vi "LJM_eNames2D.vi"(0 "Handle In":i32, 1 "NumFrames (Auto-Detect)":i32=-1, 5 "aNames":string[](array[string]), 9 "aValuesIn":dbl[][](array[numeric]) format="%.2f", 11 "error in":errorcluster, 12 "aWrites":i32[](array[ring]) items=["Read", "Write"], 13 "aNumValues":i32[](array[numeric])) -> (4 "Handle Out":i32, 10 "aValuesOut":dbl[][](array[numeric]) format="%.2f", 14 "ErrorAddress":i32, 15 "error out":errorcluster)   [LabVIEW 2020]
panel:
  # "1/20/2015:  Default value of NumFrames changed to -1 which\nequates to Auto-Detect.  If NumFrames = -1, then the NumFrames\ncontrol is ignored and the size of aNames/aAddresses is used to\ndetermine how many frames there are."
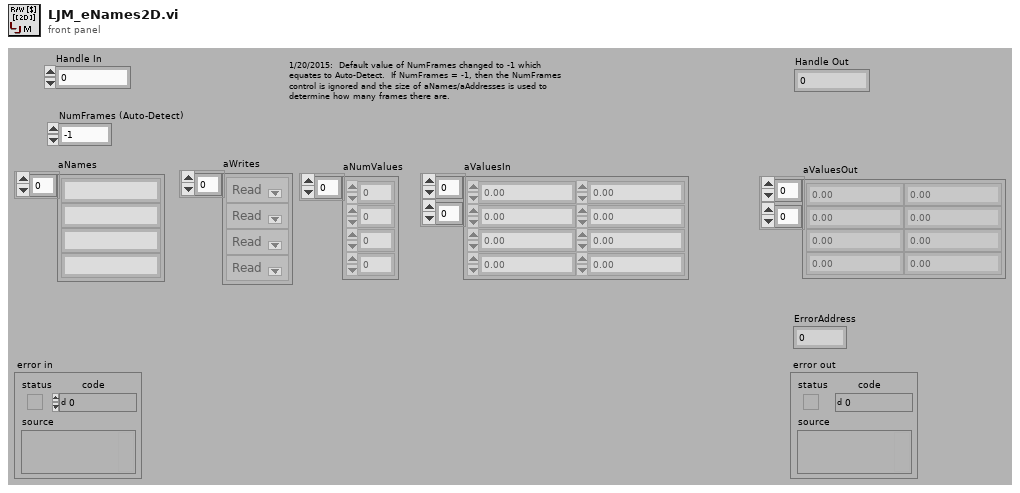
[diagram p1: front panel]
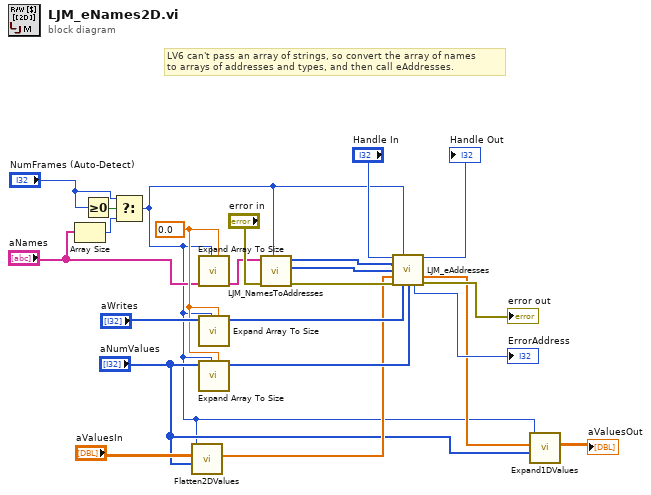
[diagram p0: block diagram]
diagram:
  w11 = 0.0 ("Default Value")
  # "LV6 can't pass an array of strings, so convert the array of names\nto arrays of addresses and types, and then call eAddresses."
  n1 = Array Size(array="aNames") -> (size(s)=w6:i32)
  n2 = Greater Or Equal To 0?(x="NumFrames (Auto-Detect)") -> (x >= 0?=w5:bool)
  n3 = Select(t="NumFrames (Auto-Detect)", s=w5, f=w6) -> (s? t:f=w1:i32)
  n4 = call "Flatten2DValues.vi"("NumValues"="aNumValues", "Values 2D"="aValuesIn", "NumFrames"=w1) -> ("Values 1D"=w8:dbl[])  [unwired: 8 in]
  n5 = call "Expand Array To Size.vi"("Default Value"=w11, "# Elements"=w1, "String Array In"="aNames") -> ("String Array Out"=w21:string[])  [unwired: 4 in, 4 out]
  n6 = call "Expand Array To Size.vi"("Default Value"=w11, "# Elements"=w1, "I32 Array In"="aWrites") -> ("I32 Array Out"=w15:i32[])  [unwired: 4 in, 4 out]
  n7 = call "Expand Array To Size.vi"("Default Value"=w11, "# Elements"=w1, "I32 Array In"="aNumValues") -> ("I32 Array Out"=w14:i32[])  [unwired: 4 in, 4 out]
  n8 = call "LJM_NamesToAddresses.vi"("NumFrames (Auto-Detect)"=w1, "error in"="error in", "aNames"=w21) -> ("error out"=w20:errorcluster, "aTypes"=w16:i32[], "aAddresses"=w17:i32[])  [unwired: 6 in]
  n9 = call "LJM_eAddresses.vi"("Handle In"="Handle In", "NumFrames"=w1, "aAddresses"=w17, "aTypes"=w16, "aValuesIn"=w8, "error in"=w20, "aWrites"=w15, "aNumValues"=w14) -> ("Handle Out"=→"Handle Out":i32, "aValuesOut"=w7:dbl[], "ErrorAddress"=→"ErrorAddress":i32, "error out"=→"error out":errorcluster)  [unwired: 4 in]
  n10 = call "Expand1DValues.vi"("NumValues"="aNumValues", "Values 1D"=w7, "NumFrames"=w1) -> ("Values 2D"=→"aValuesOut":dbl[][])  [unwired: 8 in]
